vi "Generate Combinations.vi"(11 "Upper Bound":i32=6) -> (3 "Array":cluster{i32, i32, i32}[](array[cluster]))   [LabVIEW 2025]
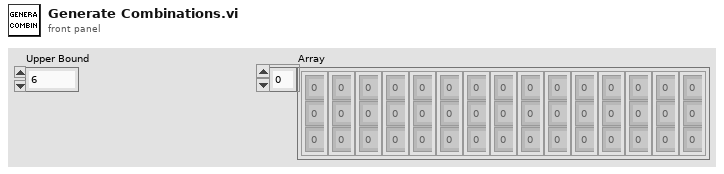
[diagram p1: front panel]
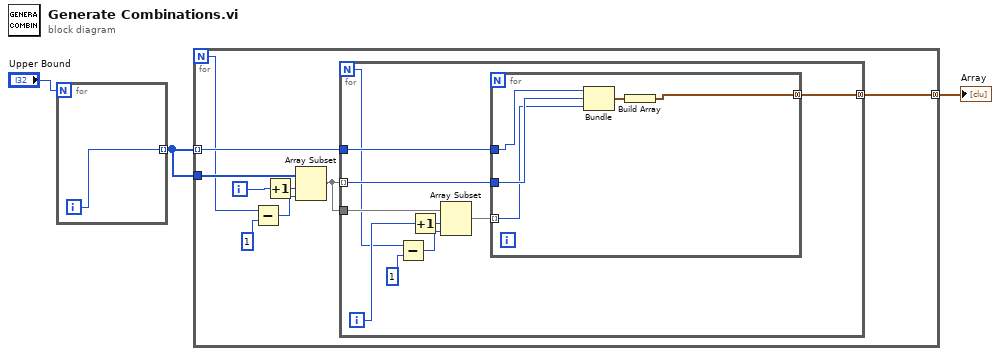
[diagram p0: block diagram]
diagram:
  n1 = for {
    N: "Upper Bound" -> [_]
    tunnel: [w4] -> w2 mode=indexing
    i -> [w4]
  }
  n2 = for {
    N -> [w8]
    tunnel: w2 -> [w13] mode=indexing
    tunnel: w2 -> [w12]
    tunnel: [w5] -> w1 mode=concatenating
    i -> [w10]
    n3 = Subtract(x=w8, y=1) -> (x-y=w9:i32)
    n4 = Increment(x=w10) -> (x+1=w11:i32)
    n5 = Array Subset(array=w12, index=w11, length=w9) -> (w6:i32[])
    n6 = for {
      N -> [w15]
      tunnel: w13 -> [w23]
      tunnel: w6 -> [w17] mode=indexing
      tunnel: w6 -> [w19]
      tunnel: [w14] -> w5 mode=concatenating
      i -> [w16]
      n7 = Subtract(x=w15, y=1) -> (x-y=w21:i32)
      n8 = Increment(x=w16) -> (x+1=w20:i32)
      n9 = Array Subset(array=w19, index=w20, length=w21) -> (w18:i32[])
      n10 = for {
        tunnel: w23 -> [w28]
        tunnel: w18 -> [w26] mode=indexing
        tunnel: w17 -> [w27]
        tunnel: [w24] -> w14 mode=concatenating
        n11 = Bundle(w28, w27, w26) -> (w25:cluster{i32, i32, i32})  [unwired: 1 in]
        n12 = Build Array(w25) -> (w24:cluster{i32, i32, i32}[])
      }
    }
  }
  "Array" <- w1
